vi "Dashboard Main.vi"() -> ()   [LabVIEW 2014]
uses:
  <vilib>/event_ctls.llb/eventvkey.ctl
  <vilib>/Rock Robotics/WPI/Dashboard/WPI_DashboardLogging Global.vi
  <vilib>/Rock Robotics/Network Tables/SD Read Number.vi
  <vilib>/Rock Robotics/Network Tables/SD Read Boolean.vi
  <vilib>/Rock Robotics/Network Tables/SD Read String.vi
  <vilib>/Utility/config.llb/Write Key (String).vi
  <vilib>/Utility/config.llb/Write Key (I32).vi
  <vilib>/Utility/config.llb/NI_LVConfig.lvlib
panel:
  in  "Rec Mode":enum32{"Stop", "Record", "Playback"}(radio)
  in  "Vision":u16(ring) items=["Camera Off", "USB Camera SW", "USB Camera HW", "IP Camera"]
  out "Camera IP":string
  out "Image Message":string="Timeout in Camera Communications"
  in  "Dashboard Tab":T1(tab)
  out "Ball Ready Shoot":bool
  out "Ball Detect":bool
  out "Shoot Down":bool
  out "Check Hot":bool
  out "Hot Goal Mimic":bool
  out "Arm State":bool=TRUE
  out "Below 60":bool
  out "PSI":dbl(slide) scale=20.0..120.0
  out "Enb":bool
  out "Ultrasonic (in)":dbl
  out "Shooter State":string="test"
  out "Run":bool
  in  "Camera Settings":T2={"Frame Rate"=30, "Compression"=30, "Size"=1} {"Frame Rate" scale=1.0..30.0; "Size" items=["640x480", "320x240", "160x120"]}
  out "MotorChart R":cluster{"Numeric":dbl, "Numeric":dbl}(graph)
  out "MotorChart L":T3(graph)
  out "MotorSliders R":cluster{"MotorSlide1":dbl, "MotorSlide2":dbl} {"MotorSlide2" scale=-1.0..1.0 scale format="%#_2e"; "MotorSlide1" scale=-1.0..1.0 scale format="%#_2e"}
  out "MotorSliders L":T4 {"MotorSlide4 2" scale=0.0..14.0 scale format="%#_2e"; "MotorSlide2" scale=-1.0..1.0 scale format="%#_2e"; "MotorSlide1" scale=-1.0..1.0 scale format="%#_2e"}
  out "Gyro":dbl(knob) scale=0.0..360.0
  out "JS1 Z":dbl(slide) scale=-1.0..1.0 scale format="%#_2e"
  out "Joystick 1":cluster{"X":dbl, "Y":dbl}[](graph)
  out "JS Buttons 1":T5
  out "JS2 Z":dbl(slide) scale=-1.0..1.0 scale format="%#_2e"
  out "Joystick 2":cluster{"X":dbl, "Y":dbl}[](graph)
  out "JS Buttons 2":T5
  out "Mode":T6(ring)=enum."Auto Disabled"
  in  "DB Camera Config":bool
  out "fps":dbl format="%#.1g"
  out "Mbps":dbl format="%#.1g"
  out "Mbps 2":bool
  in  "DB/String 9":string
  in  "DB/String 8":string
  in  "DB/String 7":string
  in  "DB/String 6":string
  in  "DB/String 5":string
  in  "DB/String 4":string
  in  "DB/String 3":string
  in  "DB/String 2":string
  in  "DB/String 1":string
  in  "DB/String 0":string
  in  "DB/Slider 0":dbl(slide) scale=0.0..5.0
  in  "DB/Slider 1":dbl(slide) scale=0.0..5.0
  in  "DB/Slider 2":dbl(slide) scale=0.0..5.0
  in  "DB/Slider 3":dbl(slide) scale=0.0..5.0
  out "DB/LED 3":bool
  out "DB/LED 2":bool
  out "DB/LED 1":bool
  out "DB/LED 0":bool
  in  "DB/Button 3":bool
  in  "DB/Button 2":bool
  in  "DB/Button 1":bool
  in  "DB/Button 0":bool
  out "Halo Sensitivity":dbl=0.75
  out "Auto To Run":dbl
  out "DB/String 10":string caption="DB/String 4"
  out "DB/String 13":string caption="DB/String 4"
  out "DB/String 12":string caption="DB/String 4"
  out "DB/String 11":string caption="DB/String 4"
  in  "Test Slider":dbl(slide) scale=0.0..100.0 scale format="%#_3g"
  in  "On/Off":bool caption="Solenoid"
  in  "Test Name":u16(ring) items=["Select the test to run...", "Example Test", "-------------------------------", "List of tests is built in robot code.", "Replace with your own automated tests."]
  in  "Test Tree":string(tree)
  in  "Motor":cluster{"Value":dbl, "Enable":bool} {"Value" scale=-1.0..1.0 scale format="%#_3g"}
  out "Progress":T7 {"Test Progress" scale=0.0..100.0}
  in  "Rev/Fwd":cluster{"Forward":bool, "Reverse":bool}
  in  "Test Ring":u16(ring) items=["Monochrome", "Color"]
  in  "Listbox":i32(listbox)
  out "Tree":string(tree)
  out "Camera Image":T8(plugin-control)
  out "Boolean":bool
  # "Left"
  # "Front"
  # "Right"
  # "True = Down\nFalse = Up"
  # "Battery"
  # "BeeScript Message Center"
  # "0 = 2 Ball \n1 = 1 Ball Hot (Move then Wait)\n2 = 1 Ball Hot (Wait then Move)\n3 = 1 Ball Hot (Wait then Move)\n4 = No shot (Wait 3  Drive 8')"
  # "Increment with Back,\nDecrement with Start."
  # "You need to Press and Hold for 1 second to make Adjustments . \n\nOnly works when Robot is Disabled."
  # "Increment with Right Bumper\nDecrement with Left Bumper"
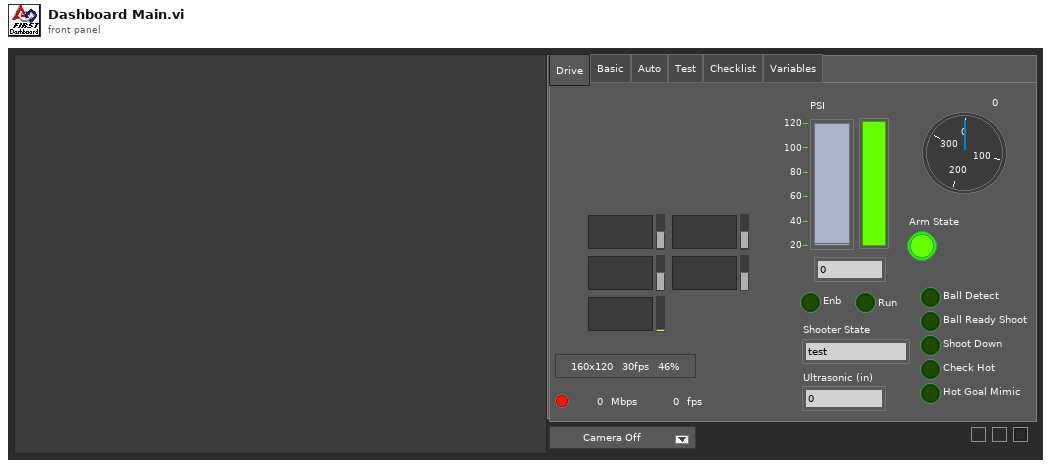
[diagram p1: front panel]
types:
  T1 = enum32{"Drive", "Basic", "Auto", "Test", "Checklist", "Variables"}
  T2 = cluster{"Frame Rate":i32, "Compression":i32, "Size":u16}
  T3 = cluster{"Numeric":dbl, "Numeric":dbl, "Battery":sgl}
  T4 = cluster{"MotorSlide1":dbl, "MotorSlide2":dbl, "MotorSlide4 2":dbl}
  T5 = cluster{bool, bool, bool, bool, bool, bool, bool, bool, bool, bool, bool, bool}
  T6 = enum8{"Tele-Op Disabled", "Tele-Op Enabled", "Auto Disabled", "Auto Enabled", "Test Disabled", "Test Enabled", ""}
  T7 = cluster{"Test Progress":u8, "Test Progress Text":string}
  T8 = typedef "IMAQ Image.ctl" = refnum<image>
  T9 = enum32{"Drive", "Basic", "Custom", "Test", "Checklist", "Variables"}
  T10 = typedef "Image Type" = u32
  T11 = cluster{"Camera Image":refnum<vi>, "Dashboard Tab":refnum<vi>, "Boolean":refnum<vi>, "Vision":refnum<vi>, "Rec Mode":refnum<vi>, "Test Slider":refnum<vi>, "On/Off ":refnum<vi>, "Test Ring":refnum<vi>, "Rev/Fwd":refnum<vi>, "Test Name":refnum<vi>, "Motor":refnum<vi>, "Progress":refnum<vi>, "CheckList":refnum<vi>, "Tree":refnum<vi>, "Test Tree":refnum<vi>}
  T12 = cluster{"Digital Inputs":bool[], "Digital Outputs":bool[]}
  T13 = cluster{"Competition mode":bool, "Robot Link":bool, "Autonomous":bool, "Enabled":bool, "E-Stop":bool, "Simulated":bool, "TestMode":bool, "Docked Window":bool}
  T14 = cluster{"Boolean Array[0]":bool, "Boolean Array[1]":bool, "Boolean Array[2]":bool, "Boolean Array[3]":bool, "Boolean Array[4]":bool, "Boolean Array[5]":bool, "Boolean Array[6]":bool, "Boolean Array[7]":bool, "Boolean Array[8]":bool, "Boolean Array[9]":bool, "Boolean Array[10]":bool, "Boolean Array[11]":bool}
  T15 = typedef "NI_LVConfig.lvlib/Config Data RefNum.ctl" = refnum<k1>
  T16 = typedef "eventvkey.ctl" = enum16{"ASCII", "Enter", "Return", "Shift", "Ctrl", "Alt", "Cmd", "Opt", "Caps", "NumLock", "Clear", "Break", "Up", "Down", "Left", "Right", "Insert", "Delete", "Home", "End", "PageUp", "PageDown", "Escape", "Help", "Pause", "ScrollLock", "F1", "F2", "F3", "F4", "F5", "F6", "F7", "F8", "F9", "F10", "F11", "F12", "F13", "F14", "F15", "F16", "F17", "F18", "F19", "F20", "F21", "F22", "F23", "F24", "Play", "VolumeUp", "VolumeDown", "Mute", "Two Byte Char"}
  T17 = cluster{"Image Size":bool, "Image Type":bool, "Pixel Value":bool, "ROI Information":bool, "Zoom Factor":bool}
  T18 = enum8{"Enabled", "Disabled", "Disabled and Grayed Out"}
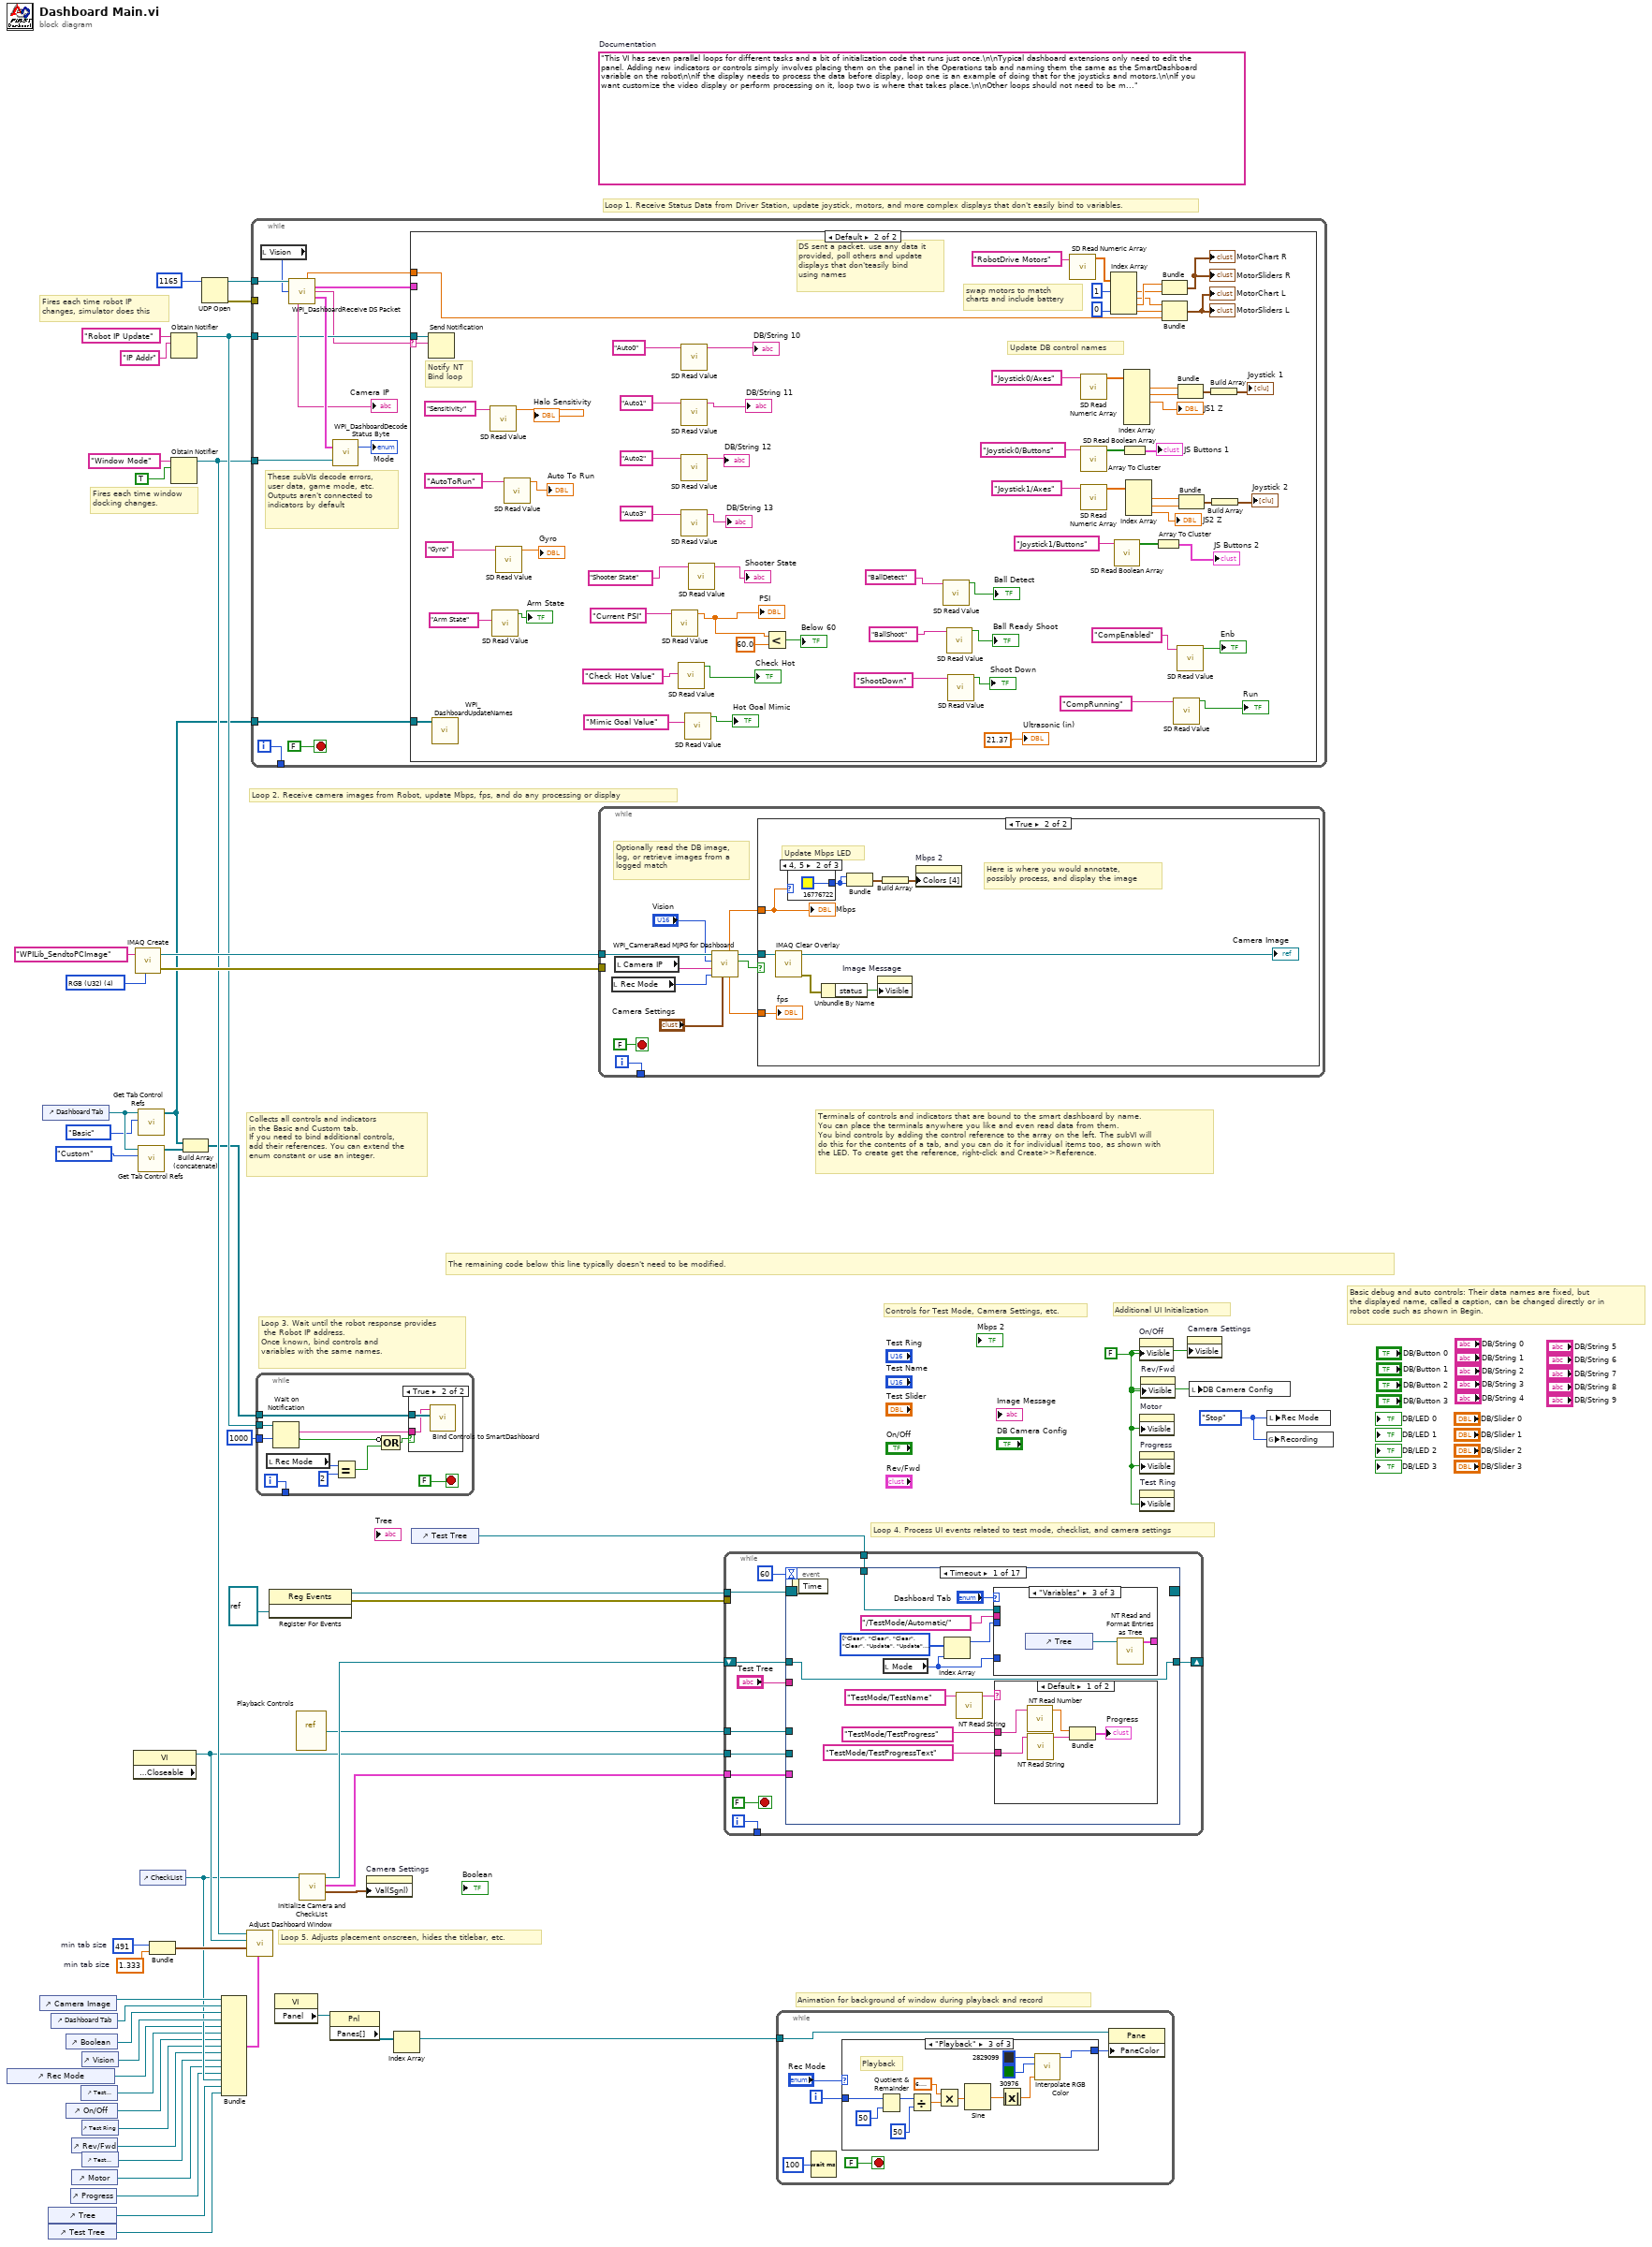
[diagram p0: block diagram]
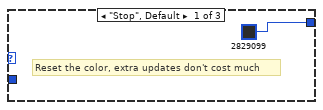
[diagram p2: hidden frame]
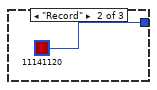
[diagram p3: hidden frame]
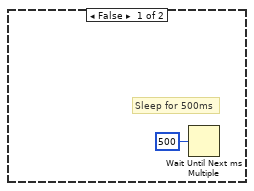
[diagram p5: hidden frame]
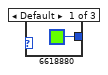
[diagram p6: hidden frame]
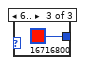
[diagram p7: hidden frame]
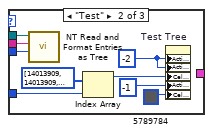
[diagram p9: hidden frame]
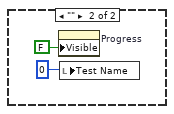
[diagram p10: hidden frame]
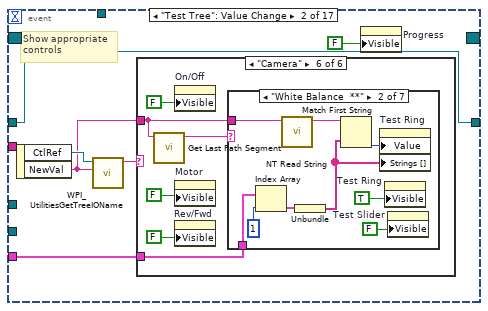
[diagram p11: hidden frame]
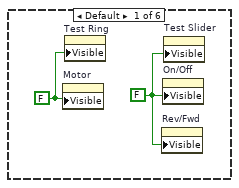
[diagram p12: hidden frame]
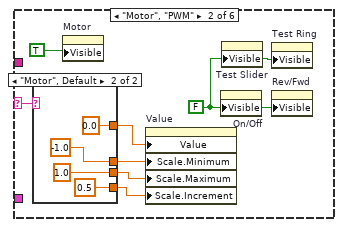
[diagram p13: hidden frame]
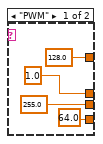
[diagram p14: hidden frame]
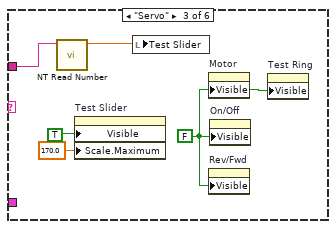
[diagram p15: hidden frame]
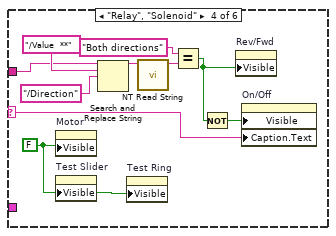
[diagram p16: hidden frame]
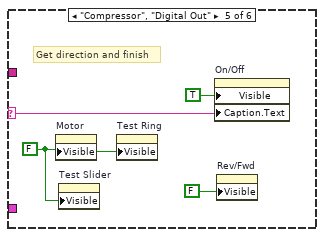
[diagram p17: hidden frame]
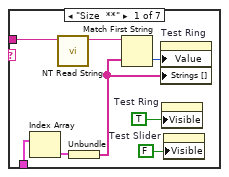
[diagram p18: hidden frame]
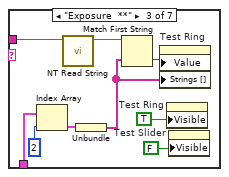
[diagram p19: hidden frame]
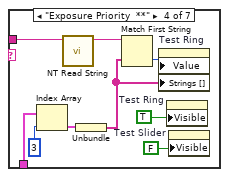
[diagram p20: hidden frame]
diagram:
  w21 = 491  # min tab size
  w20 = 1.333  # min tab size
  w29 = enum32{"Stop", "Record", "Playback"}."Stop" ("Rec Mode")
  w1 = FALSE ("Visible")
  (unwired) "This VI has seven parallel loops for different tasks and a bit of initialization code that runs just once.\n\nTypical dashboard extensions only need to edit the panel. Adding new indicators or controls simply involves placing them on the panel in the Operations tab and naming them the same as the SmartDashboard variable on the robot\n\nIf the display needs to process the data before display, loop one is an example of doing that for the joysticks and motors.\n\nIf you want customize the video display or perform processing on it, loop two is where that takes place.\n\nOther loops should not need to be modified. They are pretty standard, and document the task they perform."  # Documentation
  w51 = T10 4 items=["Grayscale (U8)", "Grayscale (I16)", "Grayscale (SGL)", "Complex (CSG)", "RGB (U32)", "HSL (U32)", "RGB (U64)"] ("Image Type")
  # "Basic debug and auto controls: Their data names are fixed, but\nthe displayed name, called a caption, can be changed directly or in\nrobot code such as shown in Begin."
  # "Controls for Test Mode, Camera Settings, etc."
  # "Additional UI Initialization"
  # "Animation for background of window during playback and record"
  # "Fires each time robot IP\nchanges, simulator does this"
  # "Fires each time window\ndocking changes."
  # "Collects all controls and indicators\nin the Basic and Custom tab.\nIf you need to bind additional controls,\nadd their references. You can extend the\nenum constant or use an integer."
  # "The remaining code below this line typically doesn't need to be modified."
  # "Loop 4. Process UI events related to test mode, checklist, and camera settings"
  # "Terminals of controls and indicators that are bound to the smart dashboard by name.\nYou can place the terminals anywhere you like and even read data from them.\nYou bind controls by adding the control reference to the array on the left. The subVI will\ndo this for the contents of a tab, and you can do it for individual items too, as shown with\nthe LED. To create get the reference, right-click and Create>>Reference."
  # "Loop 3. Wait until the robot response provides\n the Robot IP address.\nOnce known, bind controls and\nvariables with the same names."
  # "Loop 5. Adjusts placement onscreen, hides the titlebar, etc."
  # "Loop 1. Receive Status Data from Driver Station, update joystick, motors, and more complex displays that don't easily bind to variables."
  # "Loop 2. Receive camera images from Robot, update Mbps, fps, and do any processing or display"
  n1 = control-ref of="Rec Mode"() -> (w7:refnum<vi>)
  n2 = control-ref of="Camera Image"() -> (w24:refnum<vi>)
  n3 = control-ref of="Dashboard Tab"() -> (w27:refnum<vi>)
  n4 = control-ref of="Tree"() -> (w11:refnum<vi>)
  n5 = control-ref of="Test Tree"() -> (w10:refnum<vi>)
  n6 = control-ref of="Dashboard Tab"() -> (w23:refnum<vi>)
  n7 = control-ref of="Boolean"() -> (w18:refnum<vi>)
  n8 = control-ref of="On/Off"() -> (w5:refnum<vi>)
  n9 = control-ref of="Progress"() -> (w2:refnum<vi>)
  n10 = control-ref of="Rev/Fwd"() -> (w3:refnum<vi>)
  n11 = control-ref of="Motor"() -> (w8:refnum<vi>)
  n12 = control-ref of="Test Slider"() -> (w6:refnum<vi>)
  n13 = control-ref of="Vision"() -> (w22:refnum<vi>)
  n14 = control-ref of="Test Ring"() -> (w4:refnum<vi>)
  n15 = control-ref of="Test Name"() -> (w9:refnum<vi>)
  n16 = property class="VI" props=["Front Panel.Closeable"]() -> (reference out=w28:refnum<vi>)  [unwired: 2 in, 2 out]
  n17 = call "IMAQ Create"("Image Name"="WPILib_SendtoPCImage", "Image Type"=w51) -> ("New Image"=w49:T8, "error out"=w48:errorcluster)  [unwired: 2 in, 1 out]
  n18 = call <vilib>:"Get Tab Control Refs.vi"("Page Index"=T9."Basic" ("Dashboard Tab"), "TabControl in"=w27) -> ("ControlsOnPage"=w13:refnum<vi>[])  [unwired: 9 in]
  n19 = call <vilib>:"Get Tab Control Refs.vi"("Page Index"=T9."Custom" ("Dashboard Tab"), "TabControl in"=w27) -> ("ControlsOnPage"=w26:refnum<vi>[])  [unwired: 9 in]
  n20 = control-ref of="CheckList"() -> (w12:refnum<vi>)
  n21 = Bundle("min tab size"=w21, "min tab size"=w20) -> (w19:cluster{"min tab size":i32, "min tab size":dbl})  [unwired: 1 in]
  n22 = Obtain Notifier(name (unnamed)="Robot IP Update", notification data type="IP Addr" ("name (unnamed)")) -> (notifier out=w45:refnum<notifier>)  [unwired: 2 in, 2 out]
  n23 = Obtain Notifier(name (unnamed)="Window Mode", notification data type=TRUE) -> (notifier out=w30:refnum<notifier>)  [unwired: 2 in, 2 out]
  n24 = Build Array (concatenate)(w13, w26) -> (w25:refnum<vi>[])
  n25 = UDP Open(11:u16 1165 ("port")) -> (port=w52:refnum<k16>, 0:w15:errorcluster)  [unwired: 2 in, 3 out]
  n26 = Bundle("Camera Image"=w24, "Dashboard Tab"=w23, "Boolean"=w18, "Vision"=w22, "Rec Mode"=w7, "Test Slider"=w6, "On/Off"=w5, "Test Ring"=w4, "Rev/Fwd"=w3, "Test Name"=w9, "Motor"=w8, "Progress"=w2, "CheckList"=w12, "Tree"=w11, "Test Tree"=w10) -> (w14:T11)  [unwired: 1 in]
  n27 = call "Adjust Dashboard Window.vi"("Sizing Refnums"=w14, "Size Constraints"=w19, "VI"=w28, "Notifier in"=w30) -> ()  [unwired: 8 in]
  n28 = while {
    tunnel: w52 -> [w64]
    tunnel: w45 -> [w59]
    tunnel: w30 -> [w63]
    tunnel: [w60] -> _
    tunnel: w15 -> [_]
    tunnel: w13 -> [w54]
    i -> [w60]
    stop <- FALSE stop-if-true
    # "These subVIs decode errors, user data, game mode, etc.\nOutputs aren't connected to indicators by default"
    n29 = local read "Vision"() -> (w55:u16)
    n30 = call <vilib>:"WPI_DashboardReceive DS Packet.vi"("Recv Socket"=w64, "Vision"=w55) -> ("Battery"=w57:sgl, "Driver Station"=w58:T12, "Robot IP Address"=w56:string, "Status"=w65:T13, "Camera IP Address"=→"Camera IP":string)  [unwired: 1 in, 8 out]
    n31 = call <vilib>:"WPI_DashboardDecode Status Byte.vi"("Window Mode Notifier"=w63, "Status"=w65) -> ("Mode"=→"Mode":T6)  [unwired: 1 out]
    n32 = case shown="Default" w56 {
      selector: w56 -> [_ w115]
      tunnel: w59 -> [_ w116]
      tunnel: w58 -> [_ _]
      tunnel: w57 -> [_ w114]
      tunnel: w54 -> [_ w104]
      frame "0.0.0.0" {
        # "DS not sending packets, or no robot exists yet.\nDon't poll the variables"
      }
      frame Default {
        # "Update DB control names"
        # "Notify NT\nBind loop"
        # "DS sent a packet. use any data it\nprovided, poll others and update\ndisplays that don'teasily bind\nusing names"
        # "swap motors to match\ncharts and include battery"
        n33 = Send Notification(notification=w115, notifier=w116) -> ()  [unwired: 1 in, 2 out]
        n34 = call <vilib>:"WPI_DashboardUpdateNames.vi"("Controls on Tab"=w104) -> ()  [unwired: 11 in]
        n35 = call-poly <vilib>:"SD Read Value.vi"("Name"="Sensitivity") -> ("Numeric"=→"Halo Sensitivity":dbl)  [unwired: 8 in, 2 out]
        n36 = call-poly <vilib>:"SD Read Value.vi"("Table Prefix"="Arm State" ("Name")) -> ("Boolean"=→"Arm State":bool)  [unwired: 8 in, 2 out]
        n37 = call-poly <vilib>:"SD Read Value.vi"("Name"="Gyro") -> ("Numeric"=→"Gyro":dbl)  [unwired: 8 in, 2 out]
        n38 = call-poly <vilib>:"SD Read Value.vi"("Name"="AutoToRun") -> ("Numeric"=→"Auto To Run":dbl)  [unwired: 8 in, 2 out]
        n39 = call-poly <vilib>:"SD Read Value.vi"("Name"="Current PSI") -> ("Numeric"=w83:dbl)  [unwired: 8 in, 2 out]
        "PSI" <- w83
        n40 = call-poly <vilib>:"SD Read Value.vi"("Table Prefix"="Check Hot Value" ("Name")) -> ("Boolean"=→"Check Hot":bool)  [unwired: 8 in, 2 out]
        n41 = call-poly <vilib>:"SD Read Value.vi"("Name"="Auto0") -> ("String"=→"DB/String 10":string)  [unwired: 8 in, 2 out]
        n42 = call-poly <vilib>:"SD Read Value.vi"("Name"="Auto1") -> ("String"=→"DB/String 11":string)  [unwired: 8 in, 2 out]
        n43 = call-poly <vilib>:"SD Read Value.vi"("Name"="Auto2") -> ("String"=→"DB/String 12":string)  [unwired: 8 in, 2 out]
        n44 = call-poly <vilib>:"SD Read Value.vi"("Name"="Auto3") -> ("String"=→"DB/String 13":string)  [unwired: 8 in, 2 out]
        n45 = call-poly <vilib>:"SD Read Value.vi"("Table Prefix"="Mimic Goal Value" ("Name")) -> ("Boolean"=→"Hot Goal Mimic":bool)  [unwired: 8 in, 2 out]
        n46 = call-poly <vilib>:"SD Read Value.vi"("Name"="Shooter State") -> ("String"=→"Shooter State":string)  [unwired: 8 in, 2 out]
        n47 = Less?(x=w83, y=60.0) -> (x < y?=→"Below 60":bool)
        n48 = call-poly <vilib>:"SD Read Value.vi"("Name"="BallDetect") -> ("Boolean"=→"Ball Detect":bool)  [unwired: 8 in, 2 out]
        n49 = call-poly <vilib>:"SD Read Value.vi"("Name"="BallShoot") -> ("Boolean"=→"Ball Ready Shoot":bool)  [unwired: 8 in, 2 out]
        n50 = call-poly <vilib>:"SD Read Value.vi"("Name"="ShootDown") -> ("Boolean"=→"Shoot Down":bool)  [unwired: 8 in, 2 out]
        n51 = call <vilib>:"SD Read Numeric Array.vi"("Name"="RobotDrive Motors") -> ("Numeric Array"=w113:dbl[])  [unwired: 8 in, 2 out]
        n52 = call <vilib>:"SD Read Numeric Array.vi"("Name"="Joystick0/Axes") -> ("Numeric Array"=w132:dbl[])  [unwired: 8 in, 2 out]
        n53 = call <vilib>:"SD Read Boolean Array.vi"("Name"="Joystick0/Buttons") -> ("Boolean Array"=w134:bool[])  [unwired: 8 in, 2 out]
        n54 = call <vilib>:"SD Read Numeric Array.vi"("Name"="Joystick1/Axes") -> ("Numeric Array"=w126:dbl[])  [unwired: 8 in, 2 out]
        n55 = Index Array(array=w113, index #1=1, index #4=0) -> (element #1=w109:dbl, element #2=w108:dbl, element #3=w110:dbl, element #4=w105:dbl)  [unwired: 2 in]
        n56 = call <vilib>:"SD Read Boolean Array.vi"("Name"="Joystick1/Buttons") -> ("Boolean Array"=w125:bool[])  [unwired: 8 in, 2 out]
        n57 = Array To Cluster(array=w134) -> (cluster=→"JS Buttons 1":T14)
        n58 = Index Array(array=w132) -> (element #1=w129:dbl, element #2=w130:dbl, element #3=→"JS1 Z":dbl)  [unwired: 6 in, 3 out]
        n59 = Index Array(array=w126) -> (element #1=w121:dbl, element #2=w120:dbl, element #3=→"JS2 Z":dbl)  [unwired: 3 in]
        n60 = Array To Cluster(array=w125) -> (cluster=→"JS Buttons 2":T14)
        n61 = Bundle("Numeric"=w110, "Numeric"=w109) -> (→"MotorChart R" →"MotorSliders R":cluster{"Numeric":dbl, "Numeric":dbl})  [unwired: 1 in]
        n62 = Bundle("Numeric"=w108, "Numeric"=w105, "Battery"=w114) -> (→"MotorChart L" →"MotorSliders L":T3)  [unwired: 1 in]
        n63 = call-poly <vilib>:"SD Read Value.vi"("Name"="CompRunning") -> ("Boolean"=→"Run":bool)  [unwired: 8 in, 2 out]
        n64 = call-poly <vilib>:"SD Read Value.vi"("Name"="CompEnabled") -> ("Boolean"=→"Enb":bool)  [unwired: 8 in, 2 out]
        n65 = Bundle("Numeric"=w129, "Numeric"=w130) -> (w128:cluster{"Numeric":dbl, "Numeric":dbl})  [unwired: 1 in]
        n66 = Bundle("Numeric"=w121, "Numeric"=w120) -> (w122:cluster{"Numeric":dbl, "Numeric":dbl})  [unwired: 1 in]
        n67 = Build Array(w128) -> (→"Joystick 1":cluster{"Numeric":dbl, "Numeric":dbl}[])
        n68 = Build Array(w122) -> (→"Joystick 2":cluster{"Numeric":dbl, "Numeric":dbl}[])
        "Ultrasonic (in)" <- 21.37 ("Ultrasonic (in)")
      }
    }
  }
  n69 = while {
    tunnel: w25 -> [w148]
    tunnel: w45 -> [w146]
    tunnel: [w144] -> _
    tunnel: u32 1000 ("milliseconds to wait") -> [w143]
    i -> [w144]
    stop <- FALSE stop-if-true
    n70 = local read "Rec Mode"() -> (w139:enum32{"Stop", "Record", "Playback"})
    n71 = Wait on Notification(notifier=w146, timeout in ms (-1)=w143) -> (notification=w145:string, timed out?=w141:bool)  [unwired: 2 in, 2 out]
    n72 = Equal?(x=w139, y=u16 2 ("Rec Mode")) -> (x = y?=w140:bool)
    n73 = Compound Arithmetic op=OR(invert w141, w140) -> (w142:bool)
    n74 = case shown="True" w142 {
      tunnel: w148 -> [_ w150]
      tunnel: w145 -> [_ w149]
      frame False {
      }
      frame True {
        n75 = call <vilib>:"Bind Controls to SmartDashboard.vi"("Bound Control Refs"=w150, "Server IP Address"=w149) -> ()  [unwired: 10 in]
      }
    }
  }
  n76 = register-events(refnum<vi> refnum) -> (reference out=w34:refnum<event-registration>, error out=w33:errorcluster)  [unwired: 2 in]
  n77 = property class="VI"() -> ("Panel"=w37:refnum<vi>)  [unwired: 2 in, 2 out]
  n78 = vi-ref "Playback Controls.vi"() -> (w35:refnum<vi>)
  n79 = call "Initialize Camera and CheckList.vi"("ListBox in"=w12) -> ("Cluster"=w41:cluster{"value":i32, "value":i32, "index":i32}, "Array"=w42:cluster{string[]}[], "File Refnum"=w40:T15)  [unwired: 8 in]
  n80 = property class="Pnl"(reference=w37) -> ("Panes[]"=w38:refnum<vi>[])  [unwired: 1 in, 2 out]
  n81 = property on="Camera Settings" class="Clust (strict)"("Val(Sgnl)"=w41) -> ()  [unwired: 2 in, 2 out]
  n82 = Index Array(array=w38) -> (element=w36:refnum<vi>)  [unwired: 1 in]
  n83 = control-ref of="Test Tree"() -> (w39:refnum<vi>)
  n84 = while {
    tunnel: w49 -> [w159]
    tunnel: w48 -> [_]
    tunnel: [w160] -> _
    i -> [w160]
    stop <- FALSE stop-if-true
    # "Optionally read the DB image,\nlog, or retrieve images from a\nlogged match"
    n85 = local read "Rec Mode"() -> (w153:enum32{"Stop", "Record", "Playback"})
    n86 = local read "Camera IP"() -> (w151:string)
    n87 = call <vilib>:"WPI_CameraRead MJPG for Dashboard.vi"("Camera Settings"="Camera Settings", "Rec Mode"=w153, "Camera IP"=w151, "Camera Mode"="Vision", "Refnum in"=w159) -> ("Active"=w157:bool, "Refnum out"=w158:T8, "FPS"=w156:dbl, "Bandwidth (Mbps)"=w155:dbl)  [unwired: 3 in]
    n88 = case shown="True" w157 {
      tunnel: w158 -> [_ w166]
      tunnel: w155 -> [_ w165]
      tunnel: w156 -> [_ w163]
      frame False {
        # "Sleep for 500ms"
        n89 = Wait Until Next ms Multiple(millisecond multiple=u32 500) -> ()  [unwired: 1 out]
      }
      frame True {
        # "Here is where you would annotate,\npossibly process, and display the image"
        # "Update Mbps LED"
        n90 = call "IMAQ Clear Overlay"("Image"=w166) -> ("error out"=w170:errorcluster, "Image Out"=→"Camera Image":T8)  [unwired: 2 in, 7 out]
        n91 = case shown="4, 5" w165 {
          tunnel: [u32 6618880 ("Color Box") u32 16776722 ("Color Box") u32 16716800 ("Color Box")] -> w167
          frame Default {
          }
          frame 4, 5 {
          }
          frame 6.. {
          }
        }
        n92 = Unbundle By Name(w170) -> ("status"=w171:bool)
        n93 = Bundle("Color Box"=w167, "Color Box"=w167) -> (w169:cluster{"Color Box":u32, "Color Box":u32})  [unwired: 1 out]
        n94 = property on="Image Message" class="Str"("Visible"=w171) -> ()  [unwired: 2 in, 2 out]
        n95 = Build Array(w169) -> (w168:cluster{"Color Box":u32, "Color Box":u32}[])
        n96 = property on="Mbps 2" class="Bool (strict)"("Colors [4]"=w168) -> ()  [unwired: 2 in, 2 out]
        "Mbps" <- w165
        "fps" <- w163
      }
    }
  }
  n97 = while {
    tunnel: w42 -> [w182]
    shift-right: [w181] -> _
    shift-left: w40 -> [w180]
    tunnel: [w179] -> _
    tunnel: w39 -> [w178]
    tunnel: w35 -> [w177]
    tunnel: w34 -> [w176]
    tunnel: w33 -> [_]
    tunnel: w28 -> [w175]
    i -> [w179]
    stop <- FALSE stop-if-true
    n98 = event shown="[0] Timeout" {
      selector: w176 -> [_ _ _ _ _ _ _ _ _ _ _ _ _ _ _ _ _]
      dyn-events: [_ _ _ _ _ _ _ _ _ _ _ _ _ w420 _ _ _] -> _
      timeout: u32 60 ("milliseconds to wait") -> [_ _ _ _ _ _ _ _ _ _ _ _ _ _ _ _ _]
      tunnel: w178 -> [w192 _ _ _ _ _ _ _ _ _ _ _ _ _ _ _ _]
      tunnel: "Test Tree" -> [_ _ _ _ _ _ _ _ w389 w397 w399 w403 w411 _ _ _ _]
      tunnel: w182 -> [_ w216 _ _ _ _ w353 w383 _ _ _ _ _ _ _ _ _]
      tunnel: [w186 w215 w314 w319 w327 w339 w352 w376 w388 w395 w398 w402 w410 w422 w436 w437 w447] -> w181
      tunnel: w180 -> [w186 w215 w314 w319 w327 w339 w351 w376 w388 w395 w398 w402 w410 w422 w436 w437 w447]
      tunnel: w177 -> [_ _ _ _ _ _ _ _ _ _ _ _ _ w423 _ w440 _]
      tunnel: w175 -> [_ _ _ _ _ _ _ _ _ _ _ _ _ w418 _ _ _]
      event Timeout {
        w191 = enum16{"Update", "Clear"}[] [enum."Clear", enum."Clear", enum."Clear", enum."Clear", enum."Update", enum."Update", enum."Clear"] items=["Update", "Clear"]
        n99 = event-data() -> ()  [unwired: 1 in, 1 out]
        n100 = local read "Mode"() -> (w189:T6)
        n101 = Index Array(array=w191, index=w189) -> (element=w190:enum16{"Update", "Clear"})
        n102 = call <vilib>:"NT Read String.vi"("Name"="TestMode/TestName") -> ("String"=w195:string)  [unwired: 9 in, 1 out]
        n103 = case shown="\"Variables\"" "Dashboard Tab" {
          tunnel: w192 -> [_ w205 _]
          tunnel: "/TestMode/Automatic/" ("Name Pattern") -> [_ w204 _]
          tunnel: w190 -> [_ w203 _]
          tunnel: w189 -> [_ w201 _]
          tunnel: [_ _ w207] -> _
          frame "Auto", Default {
          }
          frame "Test" {
            w200 = -2 ("Active Item:Row Number")
            n104 = call <vilib>:"NT Read and Format Entries as Tree.vi"("Operation"=w203, "Name Pattern"=w204, "Tree Refnum"=w205) -> ()  [unwired: 7 in, 2 out]
            n105 = Index Array(array=u32[] [14013909, 14013909, 14013909, 14013909, 14013909, 16777215, 14013909], index=w201) -> (element=w199:u32)
            n106 = property on="Test Tree" class="Tree (strict)"("Active Item Row Number"=w200, "ActiveColNum"=w200, "CellBG"=w199, "Active Item Row Number"=-1 ("Active Item:Row Number"), "CellBG"=u32 5789784 ("Color Box")) -> ()  [unwired: 2 in, 2 out]
          }
          frame "Variables" {
            n107 = control-ref of="Tree"() -> (w206:refnum<vi>)
            n108 = call <vilib>:"NT Read and Format Entries as Tree.vi"("Tree Refnum"=w206) -> ("Formatted Strings"=w207:cluster{"Name":string, "Value":string}[])  [unwired: 9 in, 1 out]
          }
        }
        n109 = case shown="Default" w195 {
          tunnel: "TestMode/TestProgress" ("Name") -> [w209 _]
          tunnel: "TestMode/TestProgressText" ("Name") -> [w208 _]
          frame Default {
            n110 = call <vilib>:"NT Read Number.vi"("Name"=w209) -> ("Numeric"=w210:dbl)  [unwired: 9 in, 1 out]
            n111 = call <vilib>:"NT Read String.vi"("Name"=w208) -> ("String"=w211:string)  [unwired: 9 in, 1 out]
            n112 = Bundle("Numeric"=w210, "String"=w211) -> (→"Progress":cluster{"Numeric":dbl, "String":string})  [unwired: 1 in]
          }
          frame "" {
            n113 = property on="Progress" class="Clust (strict)"("Visible"=FALSE) -> ()  [unwired: 2 in, 2 out]
            n114 = local write "Test Name"(u16 0) -> ()
          }
        }
      }
      event "Test Tree": Value Change {
        # "Show appropriate\ncontrols"
        n115 = event-data() -> ("CtlRef"=w219:refnum<vi>, "NewVal"=w217:string)  [unwired: 1 in]
        n116 = call <vilib>:"WPI_UtilitiesGetTreeIOName.vi"("NewVal"=w217, "TreeControl in"=w219) -> ("I/O Name"=w220:string)  [unwired: 9 in]
        n117 = case shown="\"Camera\"" w220 {
          selector: w220 -> [_ w227 _ w245 w254 _]
          tunnel: w217 -> [_ _ w242 w244 _ w261]
          tunnel: w216 -> [_ _ _ _ _ w260]
          frame Default {
            w222 = FALSE ("Visible")
            w221 = FALSE ("Visible")
            n118 = property on="Motor" class="Clust (strict)"("Visible"=w221) -> ()  [unwired: 2 in, 2 out]
            n119 = property on="Test Ring" class="Ring (strict)"("Visible"=w221) -> ()  [unwired: 2 in, 2 out]
            n120 = property on="Rev/Fwd" class="Clust (strict)"("Visible"=w222) -> ()  [unwired: 2 in, 2 out]
            n121 = property on="On/Off" class="Bool (strict)"("Visible"=w222) -> ()  [unwired: 2 in, 2 out]
            n122 = property on="Test Slider" class="Slide (strict)"("Visible"=w222) -> ()  [unwired: 2 in, 2 out]
          }
          frame "Motor", "PWM" {
            w228 = FALSE ("Visible")
            n123 = case shown="\"Motor\", Default" w227 {
              tunnel: [1.0 ("Value") -1.0 ("Value")] -> w226
              tunnel: [255.0 ("Value") 1.0 ("Value")] -> w225
              tunnel: [128.0 ("Value") 0.0 ("Value")] -> w224
              tunnel: [64.0 ("Value") 0.5 ("Value")] -> w223
              frame "PWM" {
              }
              frame "Motor", Default {
              }
            }
            n124 = property on="Motor" class="Clust (strict)"("Visible"=TRUE) -> ()  [unwired: 2 in, 2 out]
            n125 = property on="Value" class="Slide (strict)"("Value"=w224, "Scale.Minimum"=w226, "Scale.Maximum"=w225, "Scale.Increment"=w223) -> ()  [unwired: 2 in, 2 out]
            n126 = property on="On/Off" class="Bool (strict)"("Visible"=w228) -> ()  [unwired: 2 in, 2 out]
            n127 = property on="Test Slider" class="Slide (strict)"("Visible"=w228) -> ()  [unwired: 2 in, 2 out]
            n128 = property on="Test Ring" class="Ring (strict)"("Visible"=w228) -> ()  [unwired: 2 in, 2 out]
            n129 = property on="Rev/Fwd" class="Clust (strict)"("Visible"=w228) -> ()  [unwired: 2 in, 2 out]
          }
          frame "Servo" {
            w240 = FALSE ("Visible")
            n130 = call <vilib>:"NT Read Number.vi"("Name"=w242) -> ("Numeric"=w241:dbl)  [unwired: 9 in, 1 out]
            n131 = property on="Test Slider" class="Slide (strict)"("Visible"=TRUE, "Scale.Maximum"=170.0 ("Scale.Range:Maximum")) -> ()  [unwired: 2 in, 2 out]
            n132 = local write "Test Slider"(w241) -> ()
            n133 = property on="Motor" class="Clust (strict)"("Visible"=w240) -> ()  [unwired: 2 in, 2 out]
            n134 = property on="Rev/Fwd" class="Clust (strict)"("Visible"=w240) -> ()  [unwired: 2 in, 2 out]
            n135 = property on="On/Off" class="Bool (strict)"("Visible"=w240) -> ()  [unwired: 2 in, 2 out]
            n136 = property on="Test Ring" class="Ring (strict)"("Visible"=w240) -> ()  [unwired: 2 in, 2 out]
          }
          frame "Relay", "Solenoid" {
            w243 = FALSE ("Visible")
            n137 = property on="Motor" class="Clust (strict)"("Visible"=w243) -> ()  [unwired: 2 in, 2 out]
            n138 = property on="Test Slider" class="Slide (strict)"("Visible"=w243) -> ()  [unwired: 2 in, 2 out]
            n139 = Search and Replace String(input string=w244, search string="/Value  **", replace string="/Direction") -> (result string=w250:string)  [unwired: 5 in, 3 out]
            n140 = property on="Test Ring" class="Ring (strict)"("Visible"=w243) -> ()  [unwired: 2 in, 2 out]
            n141 = call <vilib>:"NT Read String.vi"("Name"=w250) -> ("String"=w248:string)  [unwired: 9 in, 1 out]
            n142 = Equal?(x="Both directions", y=w248) -> (x = y?=w246:bool)
            n143 = Not(x=w246) -> (.not. x?=w247:bool)
            n144 = property on="Rev/Fwd" class="Clust (strict)"("Visible"=w246) -> ()  [unwired: 2 in, 2 out]
            n145 = property on="On/Off" class="Bool (strict)"("Visible"=w247, "Caption.Text"=w245) -> ()  [unwired: 2 in, 2 out]
          }
          frame "Compressor", "Digital Out" {
            w253 = FALSE ("Visible")
            # "Get direction and finish"
            n146 = property on="Motor" class="Clust (strict)"("Visible"=w253) -> ()  [unwired: 2 in, 2 out]
            n147 = property on="Test Slider" class="Slide (strict)"("Visible"=w253) -> ()  [unwired: 2 in, 2 out]
            n148 = property on="Test Ring" class="Ring (strict)"("Visible"=w253) -> ()  [unwired: 2 in, 2 out]
            n149 = property on="On/Off" class="Bool (strict)"("Visible"=TRUE, "Caption.Text"=w254) -> ()  [unwired: 2 in, 2 out]
            n150 = property on="Rev/Fwd" class="Clust (strict)"("Visible"=FALSE) -> ()  [unwired: 2 in, 2 out]
          }
          frame "Camera" {
            n151 = call <vilib>:"Get Last Path Segment.vi"("String in"=w261) -> ("String out"=w262:string)  [unwired: 10 in]
            n152 = property on="On/Off" class="Bool (strict)"("Visible"=FALSE) -> ()  [unwired: 2 in, 2 out]
            n153 = property on="Motor" class="Clust (strict)"("Visible"=FALSE) -> ()  [unwired: 2 in, 2 out]
            n154 = property on="Rev/Fwd" class="Clust (strict)"("Visible"=FALSE) -> ()  [unwired: 2 in, 2 out]
            n155 = case shown="\"White Balance  **\"" w262 {
              tunnel: w261 -> [w268 w277 w286 w295 w304 _ w310]
              tunnel: w260 -> [w266 w274 w283 w292 w301 _ _]
              frame "Size  **" {
                n156 = Index Array(array=w266) -> (element=w265:cluster{string[]})  [unwired: 1 in]
                n157 = call <vilib>:"NT Read String.vi"("Name"=w268) -> ("String"=w267:string)  [unwired: 9 in, 1 out]
                n158 = Unbundle(w265) -> (w263:string[])
                n159 = Match First String(2:w263, 3:w267) -> (0:w264:i32)  [unwired: 1 out]
                n160 = property on="Test Ring" class="Ring (strict)"("Value"=w264, "Strings []"=w263) -> ()  [unwired: 2 in, 2 out]
                n161 = property on="Test Ring" class="Ring (strict)"("Visible"=TRUE) -> ()  [unwired: 2 in, 2 out]
                n162 = property on="Test Slider" class="Slide (strict)"("Visible"=FALSE) -> ()  [unwired: 2 in, 2 out]
              }
              frame "White Balance  **" {
                n163 = Index Array(array=w274, index=1) -> (element=w275:cluster{string[]})
                n164 = call <vilib>:"NT Read String.vi"("Name"=w277) -> ("String"=w276:string)  [unwired: 9 in, 1 out]
                n165 = Unbundle(w275) -> (w272:string[])
                n166 = Match First String(2:w272, 3:w276) -> (0:w271:i32)  [unwired: 1 out]
                n167 = property on="Test Ring" class="Ring (strict)"("Value"=w271, "Strings []"=w272) -> ()  [unwired: 2 in, 2 out]
                n168 = property on="Test Ring" class="Ring (strict)"("Visible"=TRUE) -> ()  [unwired: 2 in, 2 out]
                n169 = property on="Test Slider" class="Slide (strict)"("Visible"=FALSE) -> ()  [unwired: 2 in, 2 out]
              }
              frame "Exposure  **" {
                n170 = Index Array(array=w283, index=2) -> (element=w284:cluster{string[]})
                n171 = call <vilib>:"NT Read String.vi"("Name"=w286) -> ("String"=w285:string)  [unwired: 9 in, 1 out]
                n172 = Unbundle(w284) -> (w280:string[])
                n173 = Match First String(2:w280, 3:w285) -> (0:w281:i32)  [unwired: 1 out]
                n174 = property on="Test Ring" class="Ring (strict)"("Value"=w281, "Strings []"=w280) -> ()  [unwired: 2 in, 2 out]
                n175 = property on="Test Ring" class="Ring (strict)"("Visible"=TRUE) -> ()  [unwired: 2 in, 2 out]
                n176 = property on="Test Slider" class="Slide (strict)"("Visible"=FALSE) -> ()  [unwired: 2 in, 2 out]
              }
              frame "Exposure Priority  **" {
                n177 = Index Array(array=w292, index=3) -> (element=w293:cluster{string[]})
                n178 = call <vilib>:"NT Read String.vi"("Name"=w295) -> ("String"=w294:string)  [unwired: 9 in, 1 out]
                n179 = Unbundle(w293) -> (w289:string[])
                n180 = Match First String(2:w289, 3:w294) -> (0:w290:i32)  [unwired: 1 out]
                n181 = property on="Test Ring" class="Ring (strict)"("Value"=w290, "Strings []"=w289) -> ()  [unwired: 2 in, 2 out]
                n182 = property on="Test Ring" class="Ring (strict)"("Visible"=TRUE) -> ()  [unwired: 2 in, 2 out]
                n183 = property on="Test Slider" class="Slide (strict)"("Visible"=FALSE) -> ()  [unwired: 2 in, 2 out]
              }
              frame "Color Enable  **" {
                n184 = Index Array(array=w301, index=4) -> (element=w302:cluster{string[]})
                n185 = call <vilib>:"NT Read String.vi"("Name"=w304) -> ("String"=w303:string)  [unwired: 9 in, 1 out]
                n186 = Unbundle(w302) -> (w298:string[])
                n187 = Match First String(2:w298, 3:w303) -> (0:w299:i32)  [unwired: 1 out]
                n188 = property on="Test Ring" class="Ring (strict)"("Value"=w299, "Strings []"=w298) -> ()  [unwired: 2 in, 2 out]
                n189 = property on="Test Ring" class="Ring (strict)"("Visible"=TRUE) -> ()  [unwired: 2 in, 2 out]
                n190 = property on="Test Slider" class="Slide (strict)"("Visible"=FALSE) -> ()  [unwired: 2 in, 2 out]
              }
              frame Default {
                n191 = property on="Test Ring" class="Ring (strict)"("Visible"=FALSE) -> ()  [unwired: 2 in, 2 out]
                n192 = property on="Test Slider" class="Slide (strict)"("Visible"=FALSE) -> ()  [unwired: 2 in, 2 out]
              }
              frame "Brightness  **", "Color Level  **", "Compression  **", "FPS  **", "Sharpness  **" {
                n193 = call <vilib>:"NT Read Number.vi"("Name"=w310) -> ("Numeric"=w309:dbl)  [unwired: 9 in, 1 out]
                n194 = local write "Test Slider"(w309) -> ()
                n195 = property on="Test Slider" class="Slide (strict)"("Visible"=TRUE, "Scale.Maximum"=100.0 ("Scale.Range:Maximum")) -> ()  [unwired: 2 in, 2 out]
                n196 = property on="Test Ring" class="Ring (strict)"("Visible"=FALSE) -> ()  [unwired: 2 in, 2 out]
              }
            }
          }
        }
        n197 = property on="Progress" class="Clust (strict)"("Visible"=FALSE) -> ()  [unwired: 2 in, 2 out]
      }
      event "Test Name": Mouse Enter {
        # "Populate the ring with the list of tests"
        n198 = event-data() -> ()  [unwired: 1 in, 1 out]
        n199 = call <vilib>:"NT Read String Array.vi"("Name"="TestMode/TestList") -> ("String Array"=w318:string[])  [unwired: 9 in, 1 out]
        n200 = Build Array (concatenate)("Select the test to run...", w318) -> (w317:string[])
        n201 = property on="Test Name" class="Ring (strict)"("Strings []"=w317) -> ()  [unwired: 2 in, 2 out]
      }
      event "Test Name": Value Change {
        w320 = FALSE ("Visible")
        # "Tell the robot the test name to run"
        n202 = event-data() -> ("NewVal"=w324:u16)  [unwired: 1 in]
        n203 = property on="Test Name" class="Ring (strict)"() -> ("Strings []"=w325:string[])  [unwired: 2 in, 2 out]
        n204 = local write "Progress"(T7 {"Test Progress"=0, "Test Progress Text"=""} ("Progress")) -> ()
        n205 = Index Array(array=w325, index=w324) -> (element=w323:string)
        n206 = call <vilib>:"NT Write String.vi"("String"=w323, "Name"="TestMode/TestName") -> ()  [unwired: 9 in, 1 out]
        n207 = property on="Progress" class="Clust (strict)"("Visible"=TRUE) -> ()  [unwired: 2 in, 2 out]
        n208 = property on="Motor" class="Clust (strict)"("Visible"=w320) -> ()  [unwired: 2 in, 2 out]
        n209 = property on="Test Slider" class="Slide (strict)"("Visible"=w320) -> ()  [unwired: 2 in, 2 out]
        n210 = property on="On/Off" class="Bool (strict)"("Visible"=w320) -> ()  [unwired: 2 in, 2 out]
        n211 = property on="Rev/Fwd" class="Clust (strict)"("Visible"=w320) -> ()  [unwired: 2 in, 2 out]
        n212 = property on="Test Ring" class="Ring (strict)"("Visible"=w320) -> ()  [unwired: 2 in, 2 out]
      }
      event "Listbox": Double Click {
        n213 = event-data() -> ("PlatMods.Shift"=w328:bool, "Row"=w330:i32)  [unwired: 1 in]
        n214 = case shown="True" w328 {
          tunnel: w330 -> [w334 _]
          tunnel: 1 -> [w333 _]
          frame False {
            n215 = property on="Listbox" class="LstBox (strict)"() -> ("Item Symbols"=w332:i32[])  [unwired: 2 in, 2 out]
            n216 = Replace Array Subset(array=w332, new element=w333, index=w334) -> (w331:i32[])
            n217 = property on="Listbox" class="LstBox (strict)"("Item Symbols"=w331) -> ()  [unwired: 2 in, 2 out]
          }
          frame True {
            w335 = 0 ("Top Row")
            n218 = property on="Listbox" class="LstBox (strict)"() -> ("Number of Rows"=w337:u32)  [unwired: 2 in, 2 out]
            n219 = Initialize Array(0, w337) -> (w336:i32[])
            n220 = property on="Listbox" class="LstBox (strict)"("Top Row"=w335, "Value"=w335, "Item Symbols"=w336) -> ()  [unwired: 2 in, 2 out]
          }
        }
      }
      event "Listbox": Key Down {
        n221 = event-data() -> ("VKey"=w341:T16)  [unwired: 1 in]
        n222 = case shown="\"Left\", \"Right\"" w341 {
          selector: w341 -> [w346 _]
          tunnel: eventvkey."Left" ("VKey") -> [w344 _]
          frame "Left", "Right" {
            n223 = Equal?(x=w344, y=w346) -> (x = y?=w345:bool)
            n224 = Select(t=0, s=w345, f=1) -> (s? t:f=w347:i32)
            n225 = property on="Listbox" class="LstBox (strict)"() -> ("Item Symbols"=w350:i32[])  [unwired: 2 in, 2 out]
            n226 = Replace Array Subset(array=w350, new element=w347, index="Listbox") -> (w349:i32[])
            n227 = property on="Listbox" class="LstBox (strict)"("Item Symbols"=w349) -> ()  [unwired: 2 in, 2 out]
          }
          frame Default {
          }
        }
      }
      event "DB Camera Config": Value Change {
        n228 = event-data() -> ("NewVal"=w354:bool)  [unwired: 1 in]
        n229 = case shown="True" w354 {
          tunnel: w353 -> [w363 _]
          tunnel: [w356 w374] -> w352
          tunnel: w351 -> [w355 w374]
          frame False {
            w370 = "Camera"
            w373 = FALSE ("Visible")
            n230 = local read "Camera Settings"() -> (w362:T2)
            n231 = Index Array(array=w363) -> (element=w366:cluster{string[]})  [unwired: 1 in]
            n232 = Unbundle(w362) -> ("Frame Rate"=w361:i32, "Compression"=w360:i32, "Size"=w364:u16)
            n233 = Unbundle(w366) -> (w365:string[])
            n234 = Index Array(array=w365, index=w364) -> (element=w359:string)
            n235 = call-poly <vilib>:"Write Key.vi"("section"=w370, "value"=w359, "key"="Size", "refnum"=w355) -> ("refnum out"=w372:T15)  [unwired: 2 in, 5 out]
            n236 = call-poly <vilib>:"Write Key.vi"("section"=w370, "value"=w361, "key"="FrameRate", "refnum"=w372) -> ("refnum out"=w371:T15)  [unwired: 1 in, 6 out]
            n237 = property on="Camera Settings" class="Clust (strict)"("Visible"=w373) -> ()  [unwired: 2 in, 2 out]
            n238 = local write "DB Camera Config"(w373) -> ()
            n239 = call-poly <vilib>:"Write Key.vi"("section"=w370, "value"=w360, "key"="Compression", "refnum"=w371) -> ("refnum out"=w357:T15)  [unwired: 1 in, 6 out]
            n240 = call <vilib>:"Close Config Data.vi"("refnum"=w357) -> ("file path"=w358:path)  [unwired: 2 in, 8 out]
            n241 = call <vilib>:"Open Config Data.vi"("configuration file path"=w358) -> ("refnum"=w356:T15)  [unwired: 8 in, 2 out]
          }
          frame True {
            n242 = property on="Camera Settings" class="Clust (strict)"("Visible"=TRUE) -> ()  [unwired: 2 in, 2 out]
          }
        }
      }
      event "Camera Settings": Value Change {
        n243 = event-data() -> ("NewVal"=w387:T2)  [unwired: 1 in]
        n244 = Index Array(array=w383) -> (element=w382:cluster{string[]})  [unwired: 1 in]
        n245 = Unbundle(w387) -> ("Frame Rate"=w378:i32, "Compression"=w377:i32, "Size"=w380:u16)
        n246 = Unbundle(w382) -> (w381:string[])
        n247 = Index Array(array=w381, index=w380) -> (element=w379:string)
        n248 = Format Into String(format string="%s   %dfps   %d%%", w379, w378, w377) -> (resulting string=w384:string)  [unwired: 2 in, 1 out]
        n249 = Build Array(w384) -> (w385:string[])
        n250 = property on="DB Camera Config" class="Bool (strict)"("Strings [4]"=w385) -> ()  [unwired: 2 in, 2 out]
      }
      event "Motor.Enable": Value Change {
        n251 = event-data() -> ("NewVal"=w393:bool)  [unwired: 1 in]
        n252 = Unbundle("Motor") -> ("Value"=w392:dbl)  [unwired: 1 out]
        n253 = Select(t=w392, s=w393, f=0.0) -> (s? t:f=w390:dbl)
        n254 = call <vilib>:"NT Write Number.vi"("Numeric"=w390, "Name"=w389) -> ()  [unwired: 9 in, 1 out]
      }
      event "Test Slider": Value Change {
        n255 = event-data() -> ("NewVal"=w396:dbl)  [unwired: 1 in]
        n256 = call <vilib>:"NT Write Number.vi"("Numeric"=w396, "Name"=w397) -> ()  [unwired: 9 in, 1 out]
      }
      event "On/Off": Value Change {
        n257 = event-data() -> ("NewVal"=w401:bool)  [unwired: 1 in]
        n258 = Boolean To (0,1)(Boolean=w401) -> (0, 1=w400:i16)
        n259 = call <vilib>:"NT Write Number.vi"("Numeric"=w400, "Name"=w399) -> ()  [unwired: 9 in, 1 out]
      }
      event "Rev/Fwd": Value Change {
        n260 = event-data() -> ("NewVal.Forward"=w409:bool, "NewVal.Reverse"=w408:bool)  [unwired: 1 in]
        n261 = Boolean To (0,1)(Boolean=w409) -> (0, 1=w405:i16)
        n262 = Boolean To (0,1)(Boolean=w408) -> (0, 1=w407:i16)
        n263 = Negate(x=w407) -> (-x=w406:i16)
        n264 = Add(x=w405, y=w406) -> (x+y=w404:i16)
        n265 = call <vilib>:"NT Write Number.vi"("Numeric"=w404, "Name"=w403) -> ()  [unwired: 9 in, 1 out]
      }
      event "Test Ring": Value Change {
        n266 = event-data() -> ("NewVal"=w413:u16)  [unwired: 1 in]
        n267 = property on="Test Ring" class="Ring (strict)"() -> ("Strings []"=w414:string[])  [unwired: 2 in, 2 out]
        n268 = Index Array(array=w414, index=w413) -> (element=w412:string)
        n269 = call <vilib>:"NT Write String.vi"("String"=w412, "Name"=w411) -> ()  [unwired: 9 in, 1 out]
      }
      event "Rec Mode": Value Change {
        # "Update globals for recording mode and path to read log from.\nClear when logging and let NetworkTables set path for vision to\nuse."
        n270 = event-data() -> ("NewVal"=w424:enum32{"Stop", "Record", "Playback"})  [unwired: 1 in]
        n271 = global write "WPI_DashboardLogging Global.vi" "Logging Filename"(path "") -> ()
        n272 = case shown="\"Playback\"" w424 {
          tunnel: w423 -> [_ w426 w434]
          tunnel: [_ _ w433] -> w420
          tunnel: [_ _ w432] -> _
          tunnel: w418 -> [_ _ w430]
          tunnel: cluster{i32, i32} {-250, 170} -> [_ _ w429]
          tunnel: [_ _ T17 {"Image Size"=TRUE, "Image Type"=TRUE, "Pixel Value"=TRUE, "ROI Information"=TRUE, "Zoom Factor"=FALSE} ("Image Information Shown:All Elements")] -> w416
          tunnel: [_ _ TRUE ("Zoom Factor")] -> w415
          frame Default {
          }
          frame "Stop", "Record" {
            # "Place Window too"
            n273 = invoke class="VI" method="FP.Close"(reference=w426) -> (reference out=w425:refnum<vi>)  [unwired: 2 in, 2 out]
            n274 = invoke class="VI" method="Abort VI"(reference=w425) -> ()  [unwired: 2 in, 3 out]
          }
          frame "Playback" {
            n275 = call "Open Playback Panel.vi"("Offset"=w429, "DB VI Ref"=w430, "Playback in"=w434) -> ("Playback out"=w431:refnum<vi>)  [unwired: 8 in]
            n276 = register-events(w431) -> (reference out=w433:refnum<event-registration>, error out=w432:errorcluster)  [unwired: 2 in]
          }
        }
        n277 = global write "WPI_DashboardLogging Global.vi" "Recording"(w424) -> ()
        n278 = property on="Camera Image" class="ImageControl"("Image Information Shown"=w416, "Image Information Visible"=w415) -> ()  [unwired: 2 in, 2 out]
        n279 = call <vilib>:"WPI_DashboardNT Log FieldName Cache.vi"("Operation"=enum16{"Lookup/Add", "Index", "Clear"}."Clear") -> ()  [unwired: 8 in, 3 out]
      }
      event Panel Close {
        w435 = enum32{"Stop", "Record", "Playback"}."Stop" ("Rec Mode")
        n280 = event-data() -> ()  [unwired: 1 in, 4 out]
        n281 = local write "Rec Mode"(w435) -> ()
        n282 = global write "WPI_DashboardLogging Global.vi" "Recording"(w435) -> ()
      }
      event Panel Close {
        # "Abort playback window and ourself"
        n283 = event-data() -> ()  [unwired: 1 in, 4 out]
        n284 = invoke class="VI" method="FP.Close"(reference=w440) -> (reference out=w439:refnum<vi>)  [unwired: 2 in, 2 out]
        n285 = invoke class="VI" method="Abort VI"(reference=w439) -> (error out=w438:errorcluster)  [unwired: 2 in, 2 out]
        n286 = invoke class="VI" method="Abort VI"(error in=w438) -> ()  [unwired: 2 in, 3 out]
      }
      event "Vision": Value Change {
        n287 = event-data() -> ("NewVal"=w446:u16)  [unwired: 1 in]
        n288 = Equal?(x=w446, y=u32 2 ("milliseconds to wait")) -> (x = y?=w444:bool)
        n289 = Select(t=T18."Disabled and Grayed Out" ("Disabled"), s=w444, f=T18."Enabled" ("Disabled")) -> (s? t:f=w441:T18)
        n290 = property on="Compression" class="Slide (strict)"("DisabledEnum"=w441) -> ()  [unwired: 2 in, 2 out]
      }
    }
  }
  n291 = while {
    tunnel: w36 -> [w449]
    i -> [w452]
    stop <- FALSE stop-if-true
    n292 = Wait (ms)(milliseconds to wait=u32 100) -> ()  [unwired: 1 out]
    n293 = case shown="\"Playback\"" "Rec Mode" {
      tunnel: w452 -> [_ _ w467]
      tunnel: [u32 2829099 ("Base Color") u32 11141120 ("Target Color") w456] -> w448
      frame "Stop", Default {
        # "Reset the color, extra updates don't cost much"
      }
      frame "Record" {
      }
      frame "Playback" {
        # "Playback"
        n294 = Quotient & Remainder(x=w467, y=u32 50 ("milliseconds to wait")) -> (x-y*floor(x/y)=w463:u32)  [unwired: 1 out]
        n295 = Divide(x=w463, y=u32 50 ("milliseconds to wait")) -> (x/y=w460:dbl)
        n296 = Multiply(x=6.283185307179586, y=w460) -> (x*y=w465:dbl)
        n297 = Sine(x=w465) -> (sin(x)=w464:dbl)
        n298 = Absolute Value(x=w464) -> (abs(x)=w457:dbl)
        n299 = call "Interpolate RGB Color.vi"("Proportion"=w457, "Target Color"=u32 30976, "Base Color"=u32 2829099) -> ("Result Color"=w456:u32)  [unwired: 8 in]
      }
    }
    n300 = property class="Pane"(reference=w449, "PaneColor"=w448) -> ()  [unwired: 1 in, 2 out]
  }
  n301 = property on="On/Off" class="Bool (strict)"("Visible"=w1) -> ()  [unwired: 2 in, 2 out]
  n302 = property on="Motor" class="Clust (strict)"("Visible"=w1) -> ()  [unwired: 2 in, 2 out]
  n303 = property on="Progress" class="Clust (strict)"("Visible"=w1) -> ()  [unwired: 2 in, 2 out]
  n304 = property on="Test Ring" class="Ring (strict)"("Visible"=w1) -> ()  [unwired: 2 in, 2 out]
  n305 = property on="Rev/Fwd" class="Clust (strict)"("Visible"=w1) -> ()  [unwired: 2 in, 2 out]
  n306 = property on="Camera Settings" class="Clust (strict)"("Visible"=w1) -> ()  [unwired: 2 in, 2 out]
  n307 = local write "DB Camera Config"(w1) -> ()
  n308 = global write "WPI_DashboardLogging Global.vi" "Recording"(w29) -> ()
  n309 = local write "Rec Mode"(w29) -> ()
